vi "DecodeDataFrame.vi"(8 "ErrorIn":errorcluster, 11 "Frame":string) -> (0 "ErrorOut":errorcluster, 3 "Packets":T1[](array[typedef]))   [LabVIEW 2016]
doc: "Decode data frame in order to get measument packets and other data associated with it during implementation.\n\nIf there is an arror during processing or at the input, VI ends execution and throws error."
uses:
  FallSensor/Packet.ctl
  FallSensor/Sample.ctl
  FallSensor/Reading.ctl
  FallSensor/ReadingUnits/AccelReadingUnit.ctl
  FallSensor/ReadingUnits/GyroReadingUnit.ctl
  DecodeDataFrame/DDFDataFrameSection.ctl
  DecodeDataFrame/DDFContext.ctl
  DecodeDataFrame/DDFDataFrameSectionsLen.ctl
  FallSensor/EventStatus.ctl
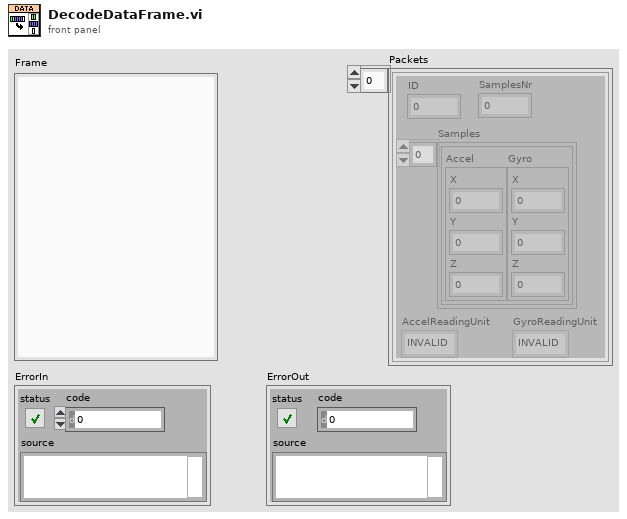
[diagram p1: front panel]
types:
  T1 = typedef "Packet.ctl" = cluster{"ID":u32, "SamplesNr":u32, "Samples":T2[], "AccelReadingUnit":T4, "GyroReadingUnit":T5}
  T2 = typedef "Sample.ctl" = cluster{"Accel":T3, "Gyro":T3}
  T3 = typedef "Reading.ctl" = cluster{"X":dbl, "Y":dbl, "Z":dbl}
  T4 = typedef "AccelReadingUnit.ctl" = enum16{"INVALID", "RAW", "g"}
  T5 = typedef "GyroReadingUnit.ctl" = enum16{"INVALID", "RAW", "°/sec"}
  T6 = typedef "DDFDataFrameSectionsLen.ctl" = cluster{"Header":i32, "PacketID":i32, "Packet":i32, "Sample":i32}
  T7 = typedef "DDFContext.ctl" = cluster{"Frame":string, "FrameHeader":string, "FrameSectionsLen":T6, "Packets":T1[], "PacketsNum":u32, "MeasFreq":u32, "EventStatus":T8, "PackedIDs":u32[]}
  T8 = typedef "EventStatus.ctl" = enum16{"IDLE", "FALL", "NONE"}
  T9 = typedef "DDFDataFrameSection.ctl" = enum16{"SOF", "Header", "PacketID", "Data", "EOF"}
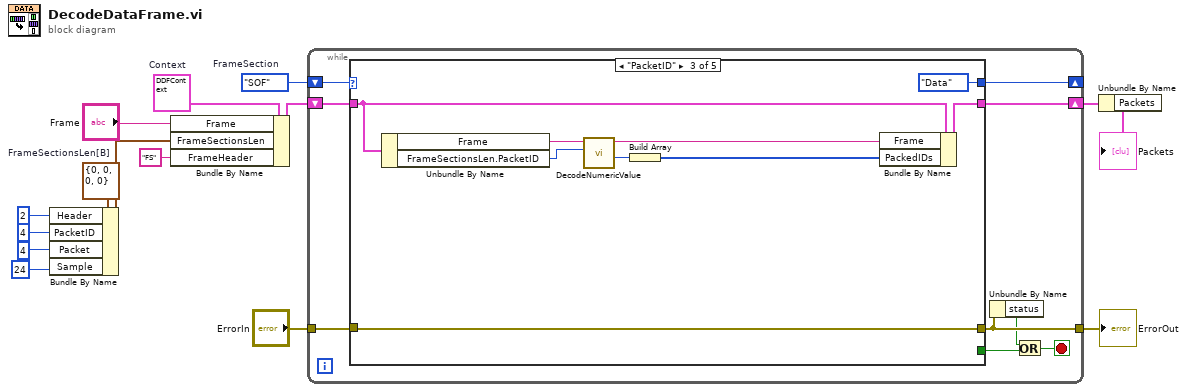
[diagram p0: block diagram]
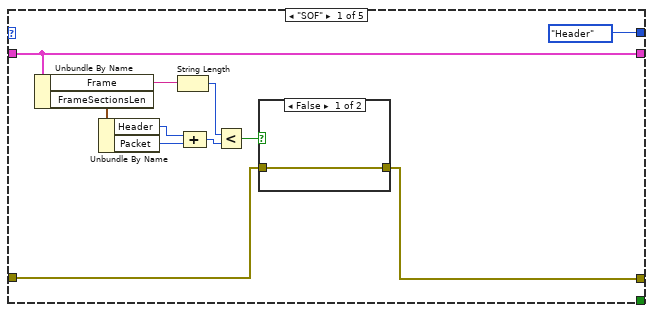
[diagram p2: hidden frame]
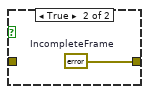
[diagram p3: hidden frame]
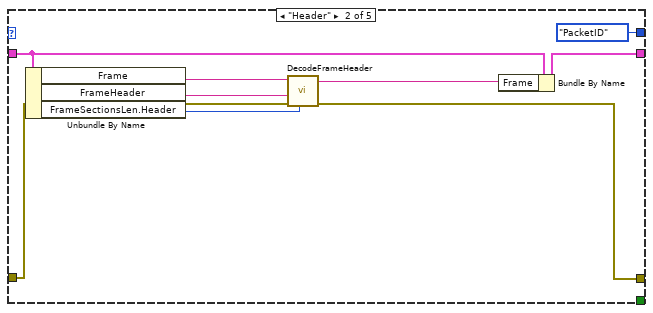
[diagram p4: hidden frame]
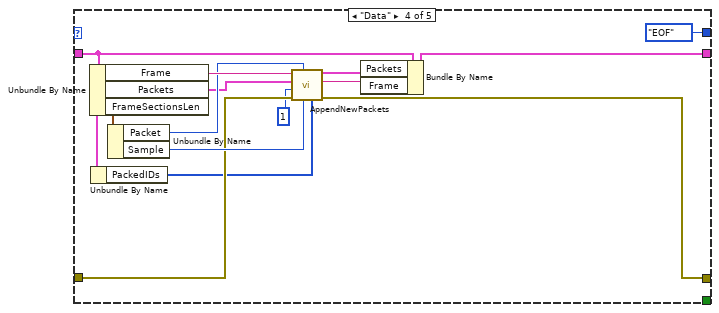
[diagram p5: hidden frame]
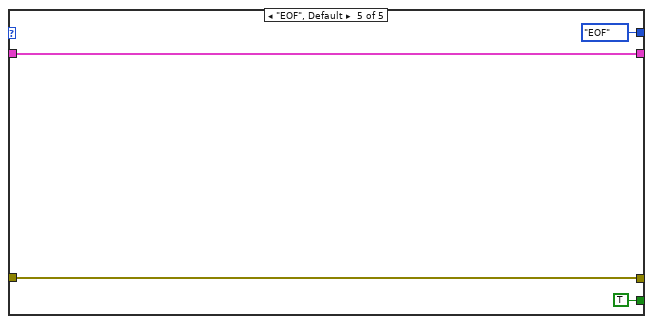
[diagram p6: hidden frame]
diagram:
  w11 = T6 {"Header"=0, "PacketID"=0, "Packet"=0, "Sample"=0}  # FrameSectionsLen[B]
  w12 = T7 {"Frame"="", "FrameHeader"="", "FrameSectionsLen"={"Header"=0, "PacketID"=0, "Packet"=0, "Sample"=0}, "Packets"=[], "PacketsNum"=0, "MeasFreq"=0, "EventStatus"=enum."IDLE", "PackedIDs"=[]}  # Context
  w1 = DDFDataFrameSection."SOF"  # FrameSection
  n1 = Bundle By Name(cluster=w11, "Header"=2, "PacketID"=4 ("PacketName"), "Packet"=4 ("Config"), "Sample"=24 ("Config")) -> (w9:T6)
  n2 = Bundle By Name(cluster=w12, "Frame"="Frame", "FrameSectionsLen"=w9, "FrameHeader"="FS") -> (w8:T7)
  n3 = while {
    shift-right: [w16] -> _
    shift-left: w1 -> [w24]
    tunnel: "ErrorIn" -> [w23]
    tunnel: [w20] -> w14
    shift-right: [w21] -> w7
    shift-left: w8 -> [w22]
    stop <- w19 stop-if-true
    n4 = case shown="\"PacketID\"" w24 {
      tunnel: [DDFDataFrameSection."Header" DDFDataFrameSection."PacketID" DDFDataFrameSection."Data" DDFDataFrameSection."EOF" DDFDataFrameSection."EOF"] -> w16
      tunnel: w23 -> [w28 w43 w52 w65 w72]
      tunnel: [w27 w42 w52 w64 w72] -> w20
      tunnel: w22 -> [w25 w45 w55 w57 w70]
      tunnel: [w25 w44 w54 w61 w70] -> w21
      tunnel: [_ _ _ _ TRUE] -> w17
      frame "SOF" {
        n5 = Unbundle By Name(w25) -> ("Frame"=w35:string, "FrameSectionsLen"=w34:T6)
        n6 = Unbundle By Name(w34) -> ("Header"=w33:i32, "Packet"=w32:i32)
        n7 = String Length(string=w35) -> (length=w31:i32)
        n8 = Compound Arithmetic op=ADD(w33, w32) -> (w30:i32)
        n9 = Less?(x=w31, y=w30) -> (x < y?=w29:bool)
        n10 = case shown="False" w29 {
          tunnel: w28 -> [w36 _]
          tunnel: [w36 w37] -> w27
          frame False {
          }
          frame True {
            w37 = errorcluster {"status"=TRUE, "code"=1, "source"="Incomplete frame"}  # IncompleteFrame
          }
        }
      }
      frame "Header" {
        n11 = Unbundle By Name(w45) -> ("Frame"=w39:string, "FrameHeader"=w38:string, "FrameSectionsLen.Header"=w41:i32)
        n12 = call "DecodeFrameHeader.vi"("HeaderLen"=w41, "ErrorIn"=w43, "Header"=w38, "Frame"=w39) -> ("ErrorOut"=w42:errorcluster, "Remainder"=w40:string)  [unwired: 5 in, 1 out]
        n13 = Bundle By Name(cluster=w45, "Frame"=w40) -> (w44:T7)
      }
      frame "PacketID" {
        n14 = Unbundle By Name(w55) -> ("Frame"=w51:string, "FrameSectionsLen.PacketID"=w50:i32)
        n15 = call "DecodeNumericValue.vi"("DataLen"=w50, "Frame"=w51) -> ("NumericValue"=w48:u32, "Remainder"=w49:string)  [unwired: 8 in]
        n16 = Build Array(w48) -> (w47:u32[])
        n17 = Bundle By Name(cluster=w55, "Frame"=w49, "PackedIDs"=w47) -> (w54:T7)
      }
      frame "Data" {
        n18 = Unbundle By Name(w57) -> ("Frame"=w68:string, "Packets"=w60:T1[], "FrameSectionsLen"=w59:T6)
        n19 = Unbundle By Name(w57) -> ("PackedIDs"=w56:u32[])
        n20 = Unbundle By Name(w59) -> ("Packet"=w67:i32, "Sample"=w66:i32)
        n21 = call "AppendNewPackets.vi"("PacketIDs"=w56, "SampleLen"=w66, "SamplesInPacketNrLen"=w67, "ErrorIn"=w65, "PacketsNum"=u32 1, "PacketsIn"=w60, "FrameIn"=w68) -> ("ErrorOut"=w64:errorcluster, "FrameOut"=w62:string, "PacketsOut"=w63:T1[])  [unwired: 2 in]
        n22 = Bundle By Name(cluster=w57, "Packets"=w63, "Frame"=w62) -> (w61:T7)
      }
      frame "EOF", Default {
      }
    }
    n23 = Unbundle By Name(w20) -> ("status"=w18:bool)
    n24 = Or(x=w18, y=w17) -> (x .or. y?=w19:bool)
  }
  "ErrorOut" <- w14
  n25 = Unbundle By Name(w7) -> ("Packets"=→"Packets":T1[])
